vi "Async Core (Actor).vi"(5 "HTTP GET Async ref":refnum<data-value>, 7 "output file":path=path "", 8 "error in (no error)":errorcluster, 9 "file size (bytes)":i64, 10 "file url":string, 11 "client handle":T1) -> ()   [LabVIEW 2019, in "HTTP Client Extensions.lvlib" / "GET Async.lvclass"]
uses:
  HTTP GET Async/GET Async.lvclass
  <vilib>/httpClient/ClientHandle.ctl
  HTTP GET Async/GET Async.lvclass/GET Async.ctl
  <vilib>/httpClient/LabVIEWHTTPClient.lvlib
panel:
  in  "Abort":bool
  out "progress":dbl(slide) scale=0.0..100.0
  out "bytes downloaded":i64
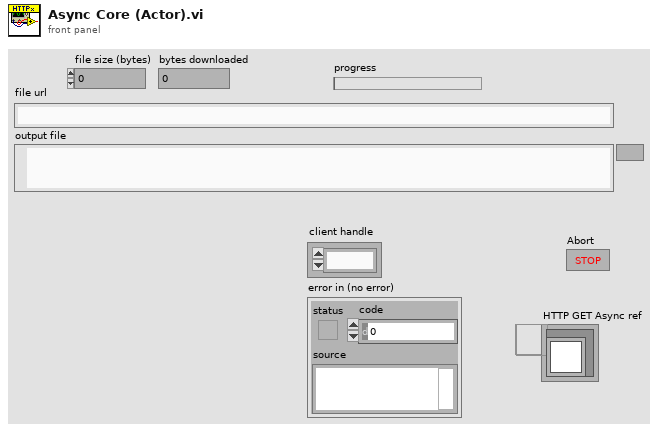
[diagram p1: front panel]
types:
  T1 = typedef "LabVIEWHTTPClient.lvlib/ClientHandle.ctl" = refnum<k1>
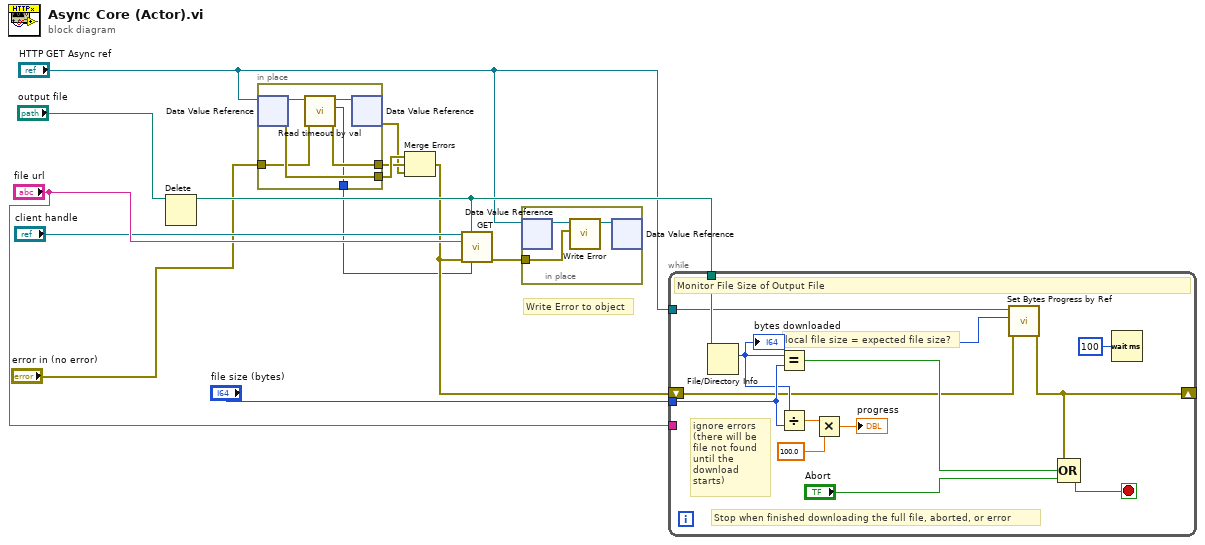
[diagram p0: block diagram]
diagram:
  # "Write Error to object"
  n1 = Delete(path (use dialog)="output file") -> (deleted path=w12:path)  [unwired: 4 in, 2 out]
  n2 = in-place {
    in-place-border: [w17] -> w7
    in-place-border: [w16] -> w8
    in-place-border: "error in (no error)" -> [w15]
    in-place-border: [w14] -> w3
    n3 = in-place-dvr #1("HTTP GET Async ref") -> (w19:refnum<class "GET Async.lvclass">, w16:errorcluster)
    n4 = call "Read timeout by val.vi"("error in (no error)"=w15, "GET Async in"=w19) -> ("error out"=w17:errorcluster, "timeout (10000)"=w14:i32, "GET Async out"=w18:refnum<class "GET Async.lvclass">)  [unwired: 7 in]
    n5 = in-place-dvr #1(w18) -> (w6:errorcluster)  [unwired: 1 out]
  }
  n6 = Merge Errors(w8, w7, w6) -> (w4:errorcluster)
  n7 = call <vilib>:"GET.vi"("client handle"="client handle", "output file"=w12, "url"="file url", "error in (no error)"=w4, "timeout (10000)"=w3) -> ("error out"=w1:errorcluster)  [unwired: 7 in, 3 out]
  n8 = in-place {
    in-place-border: w1 -> [w20]
    n9 = in-place-dvr #2("HTTP GET Async ref") -> (w22:refnum<class "GET Async.lvclass">)  [unwired: 1 out]
    n10 = call "Write Error.vi"("error"=w20, "GET Async in"=w22) -> ("GET Async out"=w21:refnum<class "GET Async.lvclass">)  [unwired: 8 in, 1 out]
    n11 = in-place-dvr #2(w21) -> ()  [unwired: 2 out]
  }
  n12 = while {
    tunnel: w12 -> [w35]
    tunnel: "file url" -> [_]
    tunnel: "file size (bytes)" -> [w32]
    shift-right: [w24] -> _
    shift-left: w4 -> [w25]
    tunnel: "HTTP GET Async ref" -> [w27]
    stop <- w30 stop-if-true
    # "ignore errors\n(there will be file not found until the download starts)"
    # "Stop when finished downloading the full file, aborted, or error"
    # "local file size = expected file size?"
    # "Monitor File Size of Output File"
    n13 = File/Directory Info(path=w35) -> (size=w26:i64)  [unwired: 1 in, 6 out]
    "bytes downloaded" <- w26
    n14 = Equal?(x=w26, y=w32) -> (x = y?=w31:bool)
    n15 = Divide(x=w26, y=w32) -> (x/y=w34:dbl)
    n16 = Multiply(x=w34, y=100.0) -> (x*y=→"progress":dbl)
    n17 = call "Set Bytes Progress by Ref.vi"("error in (no error)"=w25, "bytes downloaded"=w26, "HTTP GET Async ref in"=w27) -> ("error out"=w24:errorcluster)  [unwired: 7 in, 1 out]
    n18 = Compound Arithmetic op=OR(w24, w31, "Abort") -> (w30:bool)
    n19 = Wait (ms)(milliseconds to wait=u32 100) -> ()  [unwired: 1 out]
  }
